vi "Console.vi"(8 "error in (no error)":errorcluster) -> (0 "error out":errorcluster)   [LabVIEW 2020, in "MGI-Console.lvlib" / "Console.lvclass"]
doc: "Initialize the console.\n----\nCopyright: MGI 2018\nAuthor: Derek Trepanier"
uses:
  Console.lvclass
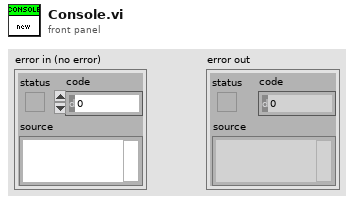
[diagram p1: front panel]
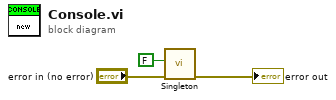
[diagram p0: block diagram]
diagram:
  n1 = call "Singleton.vi"("error in (no error)"="error in (no error)", "Close?"=FALSE) -> ("error out"=→"error out":errorcluster)  [unwired: 9 in]
